vi "Create_Temporary_Path_forPNG_and_Substitute_into_HTML.vi"(7 "offset past match":i32, 8 "error in (no error)":errorcluster, 9 "Identifying_String":string="img src=\"", 10 "SubFolderName":string="filters", 11 "Dencrypted text":string) -> (0 "error out":errorcluster, 1 "PNG_fileName":string, 2 "Temp_PATH":path, 3 "HTML_wPathChanged":string, 5 "offset past match":i32)   [LabVIEW 2016]
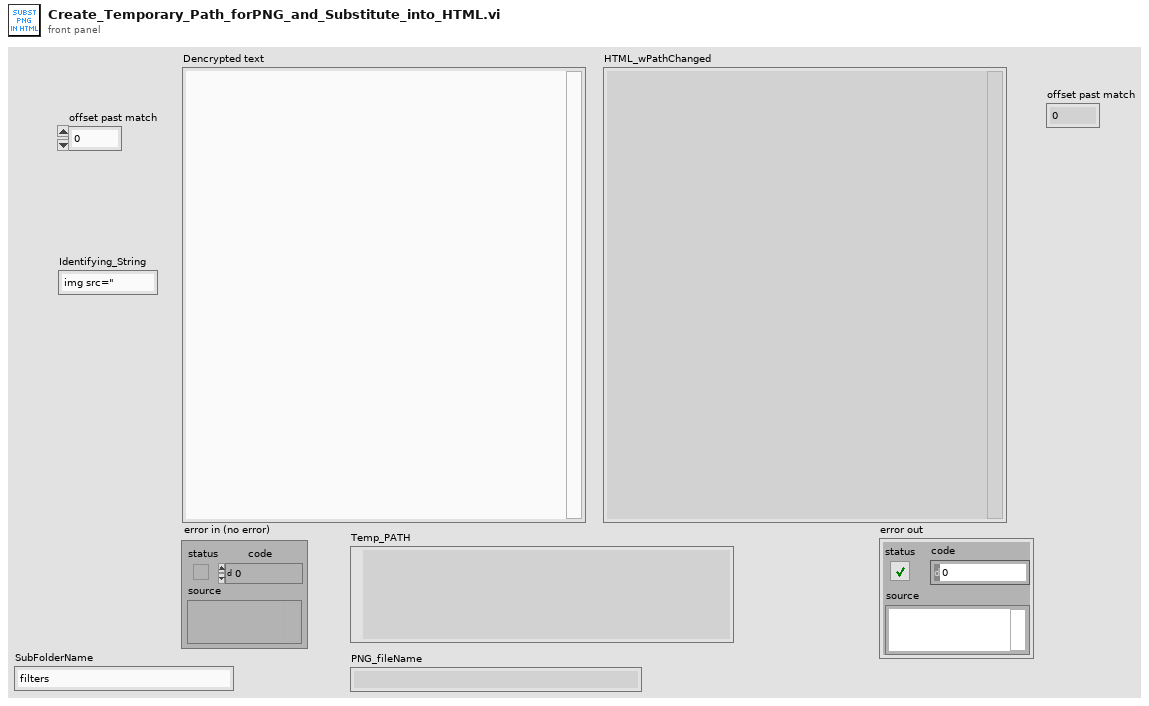
[diagram p1: front panel]
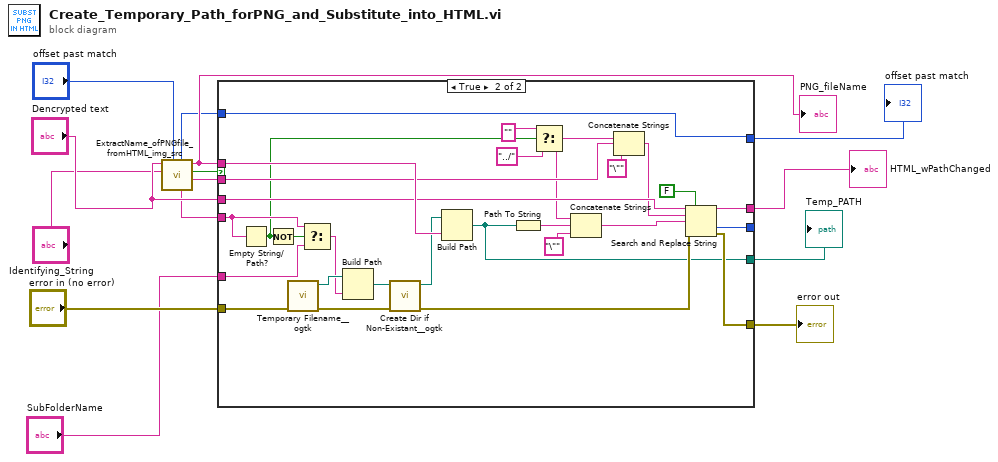
[diagram p0: block diagram]
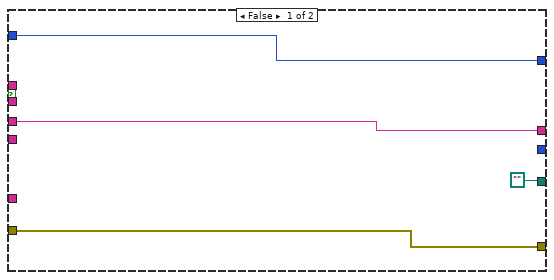
[diagram p2: hidden frame]
diagram:
  n1 = call "ExtractName_ofPNGfile_fromHTML_img_src.vi"("offset (0)"="offset past match", "Identifying_String"="Identifying_String", "Dencrypted HTML"="Dencrypted text") -> ("AllText"=w7:string, "Found?"=w6:bool, "PNG_fileName"=w14:string, "FolderName"=w1:string, "offset past match"=w5:i32)  [unwired: 3 in, 1 out]
  "PNG_fileName" <- w14
  n2 = case shown="True" w6 {
    tunnel: w14 -> [_ w46]
    tunnel: "Dencrypted text" -> [w15 w41]
    tunnel: "error in (no error)" -> [w18 w39]
    tunnel: [w15 w38] -> w11
    tunnel: [w18 w35] -> w10
    tunnel: [path "" w34] -> w9
    tunnel: w7 -> [_ w32]
    tunnel: [w17 w29] -> w4
    tunnel: w5 -> [w17 w29]
    tunnel: "SubFolderName" -> [_ w26]
    tunnel: w1 -> [_ w25]
    tunnel: [_ w19] -> _
    frame False {
    }
    frame True {
      n3 = Empty String/Path?(string/path=w25) -> (empty?=w21:bool)
      n4 = Not(x=w21) -> (.not. x?=w27:bool)
      n5 = call <userlib>:"Temporary Filename__ogtk.vi"("error in (no error)"=w39) -> ("error out"=w37:errorcluster, "file in tmp dir"=w40:path)  [unwired: 5 in]
      n6 = Select(t=w25, s=w27, f=w26) -> (s? t:f=w24:string)
      n7 = Build Path(base path=w40, name or relative path=w24) -> (appended path=w33:path)
      n8 = call <userlib>:"Create Dir if Non-Existant__ogtk.vi"("error in (no error)"=w37, "Directory Path"=w33) -> ("error out"=w36:errorcluster, "dup Directory Path"=w28:path)  [unwired: 7 in, 1 out]
      n9 = Build Path(base path=w28, name or relative path=w46) -> (appended path=w34:path)
      n10 = Path To String(path=w34) -> (string=w43:string)
      n11 = Select(t="" ("search string"), s=w21, f="../" ("search string")) -> (s? t:f=w23:string)
      n12 = Concatenate Strings(w23, w43, "\"") -> (w44:string)
      n13 = Concatenate Strings(w23, w32, "\"") -> (w30:string)
      n14 = Search and Replace String(replace all?=FALSE ("replace all? (F)"), input string=w41, search string=w30, replace string=w44, error in=w36) -> (result string=w38:string, offset past replacement=w19:i32, error out=w35:errorcluster)  [unwired: 3 in, 1 out]
    }
  }
  "HTML_wPathChanged" <- w11
  "error out" <- w10
  "Temp_PATH" <- w9
  "offset past match" <- w4
